vi "APSxSensorLoadFile.vi"(8 "error in (no error)":errorcluster caption="错误输入（无错误）", 10 "FileName":string, 11 "hSENSOR":i32) -> (0 "error out":errorcluster caption="错误输出")   [LabVIEW 2018]
doc: "该模板用于创建子VI。"
uses:
  APSx.dll/APSx.dll
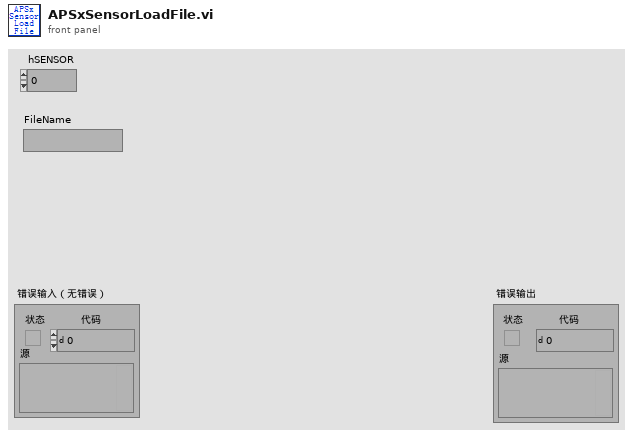
[diagram p1: front panel]
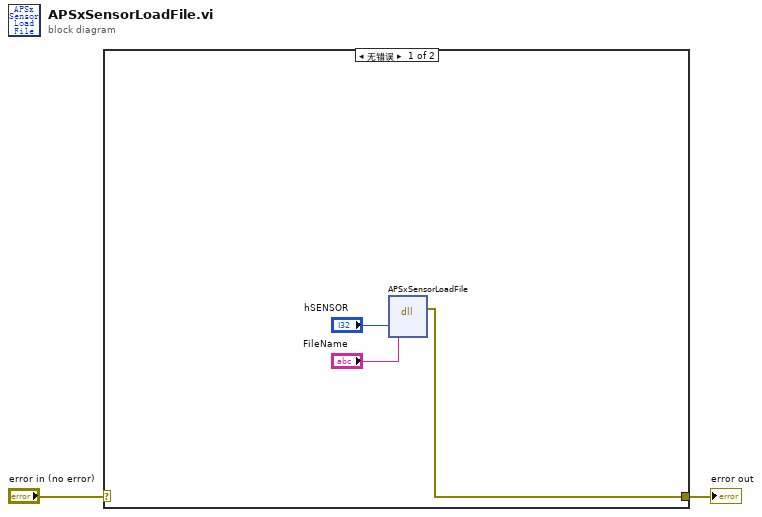
[diagram p0: block diagram]
diagram:
  n1 = case shown="无错误" "error in (no error)" {
    selector: "error in (no error)" -> [_ w6]
    tunnel: [w3 w6] -> w1
    frame No Error {
      n2 = dll-call lib="PTH2]abs D项目Feng恒隆项目Labview传感器对中台SourcesAPSx.dllAPSx.dll" fn="APSxSensorLoadFile"("hSENSOR"="hSENSOR", "FileName"="FileName") -> (error out=w3:errorcluster)  [unwired: 6 in, 1 out]
    }
    frame Error {
    }
  }
  "error out" <- w1
